vi "I2C_ReadSlaveACK_2.vi"(8 "error in":errorcluster, 10 "HalfCycle(Ticks)":u32, 11 "InterByteTransmitDelay(Ticks)":u32) -> (0 "error out":errorcluster, 3 "SDA":bool)   [LabVIEW 2019]
doc: "Yields control of the SDA line to the Slave Device and reads the Slave Device's ACK\n\n<b>Inputs:</b>\n--------------------\n<b>HalfCycle(Ticks)</b> this the number of FPGA clock cycles in half og the clock period. Therefore twice this number yields the clock period, in ticks.\n\n<b>PostAddressDelay(Ticks)</b> the delay in FPGA clock cycles before writing bytes on SDA.\n\n<b>Output</b>\n--------------------\n<b>SDA</b> value of the SDA line read in. True = slave device did not acknowledge, False = slave device acknowledged the byte writen.\n\nSee block diagram for more details on the implementation details.\n\nAuthor:\nPeter Fuller\nSenior Engineer\nPLF Consulting, LLC\n\nemail: peter@plfconsulting.com\nphone: 617.699.2201"
uses:
  <vilib>/eio/EIONode/EIONode.xnode
  Instance           1 24Saved   I2C_ReadSlaveACK .vi
  Instance           2 24Saved   I2C_ReadSlaveACK .vi
  Instance           3 24Saved   I2C_ReadSlaveACK .vi
  <vilib>/eio/EIOMethodNode/EIOMethodNode.xnode
  <vilib>/rvi/eio/common/nirviEmuTemplateMethod_errors.vi
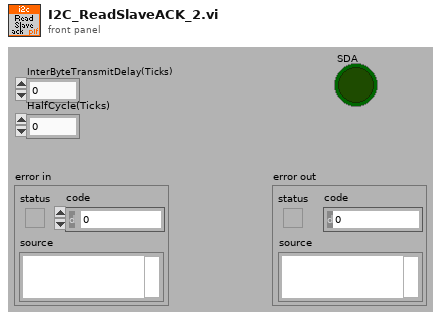
[diagram p1: front panel]
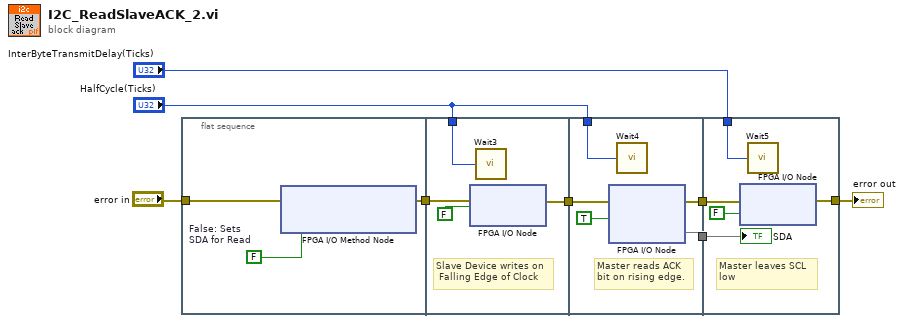
[diagram p0: block diagram]
diagram:
  n1 = flat-sequence {
    tunnel: [w10] -> w8
    tunnel: "error in" -> [w9]
    tunnel: w8 -> [w14]
    tunnel: [w13] -> w5
    tunnel: "HalfCycle(Ticks)" -> [w12]
    tunnel: [w19] -> w3
    tunnel: w5 -> [w18]
    tunnel: [w17] -> w2
    tunnel: "HalfCycle(Ticks)" -> [w16]
    tunnel: w3 -> [w22]
    tunnel: w2 -> [w24]
    tunnel: "InterByteTransmitDelay(Ticks)" -> [w21]
    tunnel: [w23] -> w6
    frame #0 {
      w11 = FALSE  # False: Sets  SDA for Read
      n2 = xnode "FPGA I/O Method Node"("error in"=w9, "Enable"=w11) -> ("error out"=w10:errorcluster)  [unwired: 1 in, 1 out]
    }
    frame #1 {
      # "Slave Device writes on\n Falling Edge of Clock"
      n3 = xnode "FPGA I/O Node"("error in"=w14, "SCL2"=FALSE ("Value")) -> ("error out"=w13:errorcluster)  [unwired: 1 in, 1 out]
      n4 = call "Wait3"("Count(Ticks)"=w12) -> ()  [unwired: 1 out]
    }
    frame #2 {
      # "Master reads ACK\nbit on rising edge."
      n5 = xnode "FPGA I/O Node"("error in"=w18, "SCL2"=TRUE ("Value")) -> ("error out"=w17:errorcluster, "SDA2"=w19)  [unwired: 2 in, 2 out]
      n6 = call "Wait4"("Count(Ticks)"=w16) -> ()  [unwired: 1 out]
    }
    frame #3 {
      # "Master leaves SCL \nlow"
      n7 = xnode "FPGA I/O Node"("error in"=w24, "SCL2"=FALSE ("Value")) -> ("error out"=w23:errorcluster)  [unwired: 1 in, 1 out]
      n8 = call "Wait5"("Count(Ticks)"=w21) -> ()  [unwired: 1 out]
      "SDA" <- w22
    }
  }
  "error out" <- w6
